vi "get enable trig out after config.vi"(8 "error in (no error)":errorcluster, 11 "LineCCD in":refnum<class "LineCCD.lvclass">) -> (0 "error out":errorcluster, 3 "LineCCD out":refnum<class "LineCCD.lvclass">)   [LabVIEW 2012, in "LineCCD.lvclass"]
uses:
  LineCCD.lvclass
  LineCCD.lvclass/LineCCD.ctl
  <instrlib>/ALPHALAS CCD S Series/ALPHALAS CCD S Series.lvlib
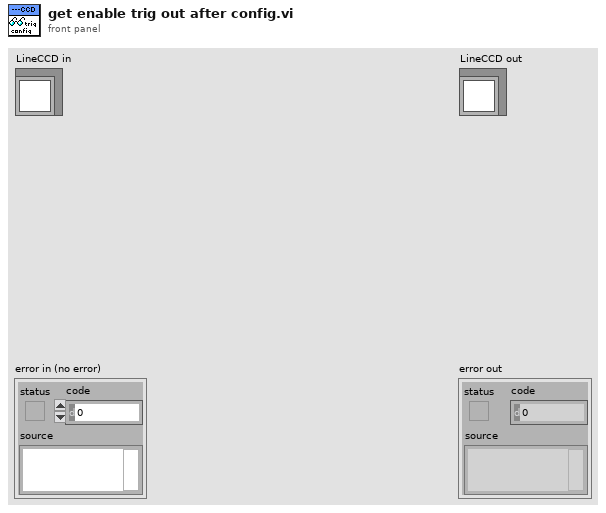
[diagram p1: front panel]
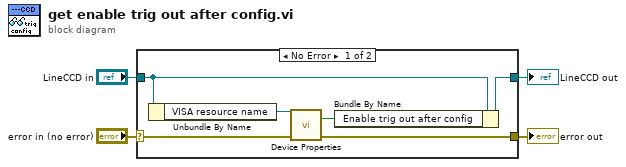
[diagram p0: block diagram]
diagram:
  n1 = case shown="No Error" "error in (no error)" {
    selector: "error in (no error)" -> [w9 w12]
    tunnel: [w8 w12] -> w3
    tunnel: [w6 w11] -> w1
    tunnel: "LineCCD in" -> [w7 w11]
    frame No Error {
      n2 = Unbundle By Name(w7) -> ("VISA resource name"=w10:refnum<visa-resource-name>)
      n3 = call <instrlib>:"Device Properties.vi"("VISA resource name"=w10, "error in (no error)"=w9) -> ("Trig Out Enabled"=w5:bool, "error out"=w8:errorcluster)  [unwired: 6 in, 18 out]
      n4 = Bundle By Name(cluster=w7, "Enable trig out after config"=w5) -> (w6:refnum<class "LineCCD.lvclass">)
    }
    frame Error {
    }
  }
  "error out" <- w3
  "LineCCD out" <- w1
